vi "Run Test Suite.vi"(8 "error in (no error)":errorcluster, 10 "Test Case":refnum<class "LUnit Test Suite.lvclass">, 11 "Execution API In":refnum<class "Execution API.lvclass">) -> (0 "error out":errorcluster, 3 "Execution API Out":refnum<class "Execution API.lvclass">)   [LabVIEW 2020, in "Execution API.lvclass"]
doc: "Run all tests in a Test Suite."
uses:
  Execution API.lvclass
  API/LUnit Test Suite/LUnit Test Suite.lvclass
  C:/git/astemes-lunit/source/Core/Runnable/Runnable.lvclass
  Execution API.lvclass/Execution API.ctl
  Framework/Test Runner/Test Runner.lvclass
  Framework/Plugin/Plugin.lvclass
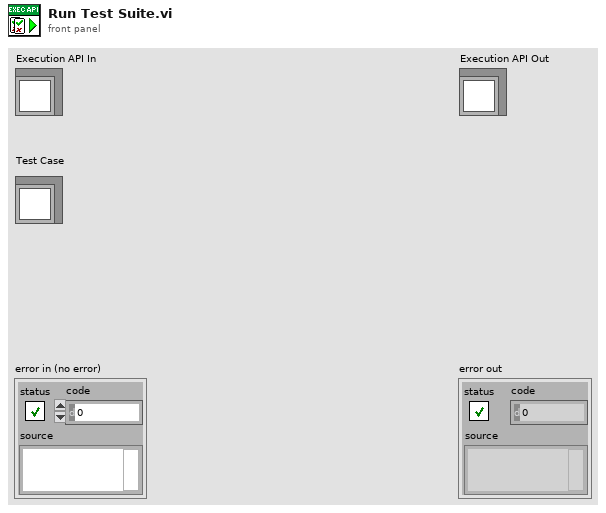
[diagram p1: front panel]
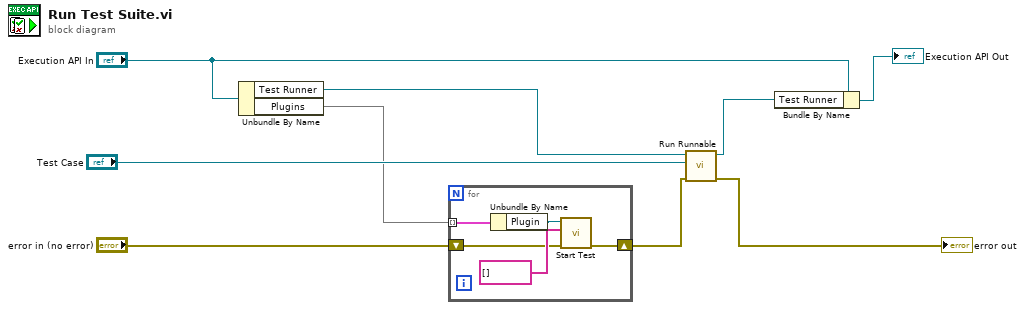
[diagram p0: block diagram]
diagram:
  n1 = Unbundle By Name("Execution API In") -> ("Test Runner"=w9:refnum<class "Test Runner.lvclass">, "Plugins"=w3:map{string, refnum<class "Plugin.lvclass">})
  n2 = for {
    tunnel: w3 -> [w14] mode=indexing
    shift-right: [w11] -> w2
    shift-left: "error in (no error)" -> [w10]
    n3 = Unbundle By Name(w14) -> ("Plugin"=w13:refnum<class "Plugin.lvclass">)
    n4 = call-dynamic "Start Test.vi"("error in (no error)"=w10, "Tests"=string[] [], "Plugin in"=w13) -> ("error out"=w11:errorcluster)  [unwired: 7 in, 1 out]
  }
  n5 = call-dynamic "Run Runnable.vi"("error in (no error)"=w2, "Runnable"="Test Case", "Test Runner In"=w9) -> ("error out"=→"error out":errorcluster, "Test Runner Out"=w8:refnum<class "Test Runner.lvclass">)  [unwired: 7 in]
  n6 = Bundle By Name(cluster="Execution API In", "Test Runner"=w8) -> (→"Execution API Out":refnum<class "Execution API.lvclass">)
